vi "N6700_PowerSupplyGUI.vi"(11 "error in (no error)":errorcluster) -> (4 "PsGuiRef":refnum<vi>, 15 "error out":errorcluster {"code" format="%.0x"})   [LabVIEW 2018]
panel:
  out "String":string caption="Timeout"
  in  "Tab Control":enum32{"Page 1", "Page 2"}(tab)
  in  "VISA session":refnum<visa-resource-name>="TCPIP0::169.254.70.130::inst0::INSTR"
  in  "Current Lim":sgl[](array[numeric])
  in  "Voltage Set":sgl[](array[numeric])
  in  "stop":bool=TRUE
  in  "STATE":bool[](array[boolean])=[FALSE, FALSE, FALSE, FALSE]
  out "Volts":dbl[](array[numeric])=[-1.0, -1.0, -1.0, -1.0]
  in  "Measure":bool
  out "Amps":dbl[](array[numeric])=[-1.0, -1.0, -1.0, -1.0]
  in  "RESET_PS":bool=TRUE
  in  "Output Couple Channels(t)":bool=TRUE
  in  "poll rate(ms)":u32=1000
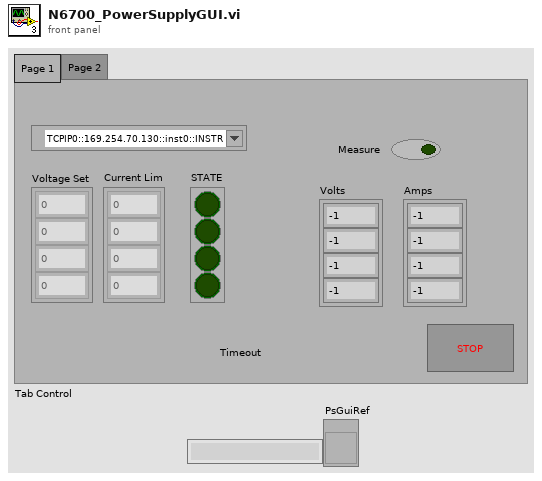
[diagram p1: front panel]
types:
  T1 = enum32{"Invalid", "Standard", "Closed", "Hidden", "Minimized", "Maximized"}
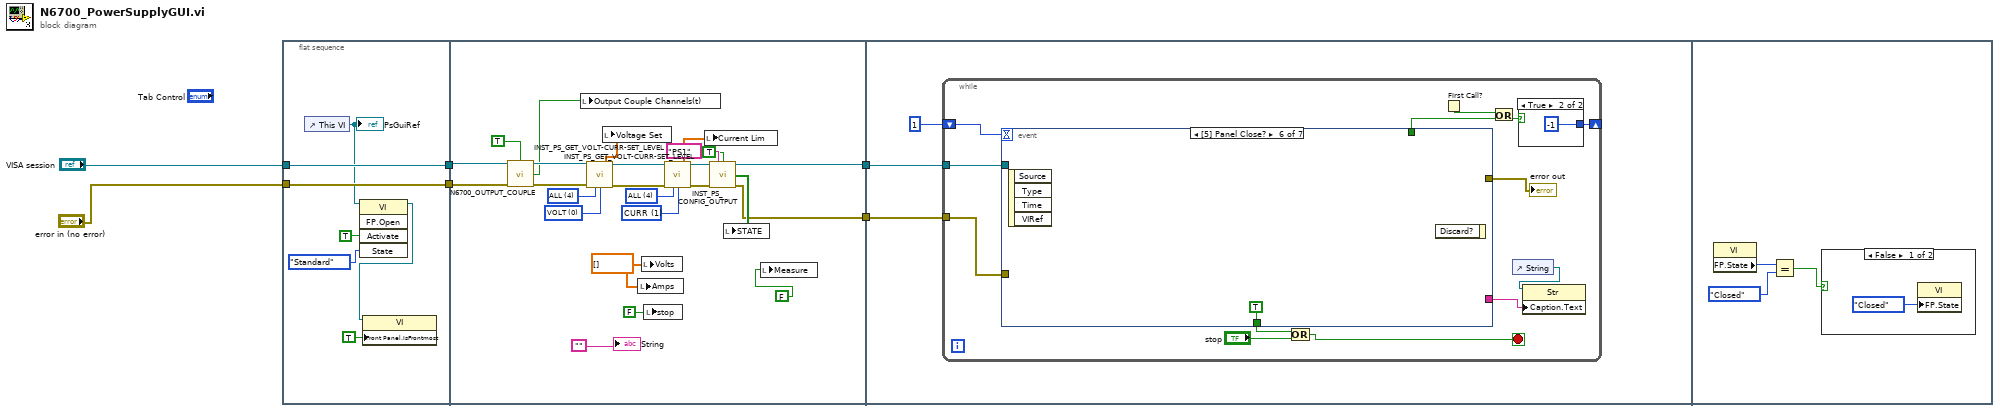
[diagram p0: block diagram]
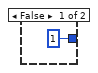
[diagram p2: hidden frame]
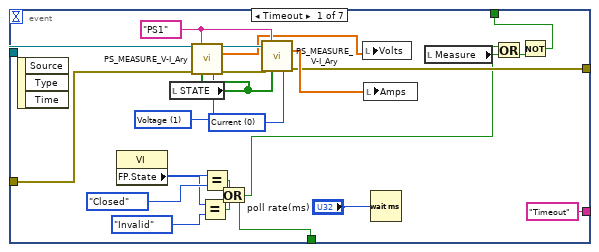
[diagram p3: hidden frame]
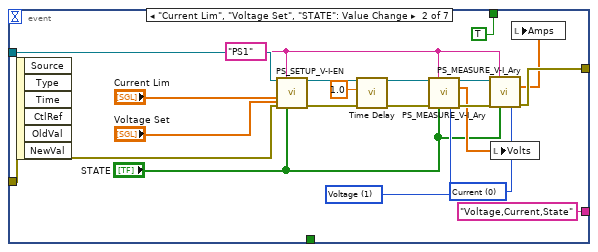
[diagram p4: hidden frame]
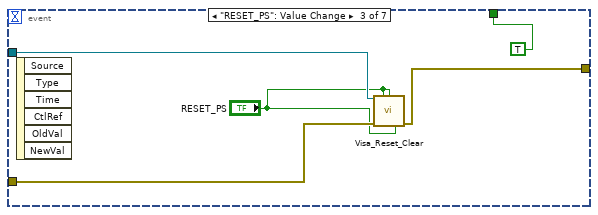
[diagram p5: hidden frame]
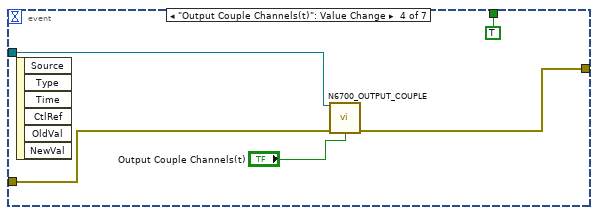
[diagram p6: hidden frame]
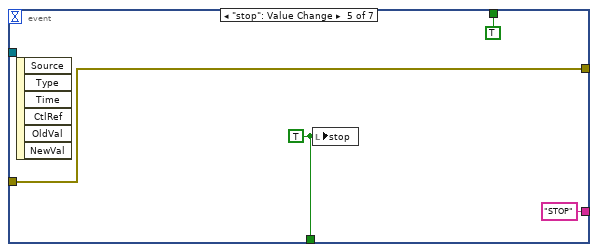
[diagram p7: hidden frame]
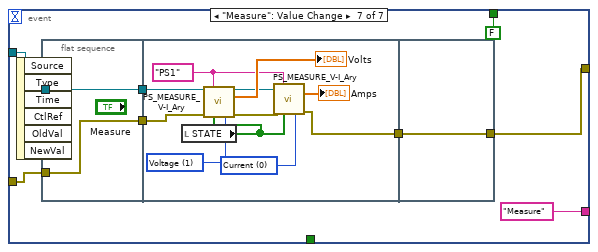
[diagram p8: hidden frame]
diagram:
  n1 = flat-sequence {
    tunnel: "error in (no error)" -> [w12]
    tunnel: "VISA session" -> [w13]
    tunnel: [w13] -> w2
    tunnel: [w12] -> w1
    tunnel: [w24] -> w5
    tunnel: [w21] -> w3
    tunnel: w2 -> [w20]
    tunnel: w1 -> [w19]
    tunnel: w5 -> [w41]
    tunnel: w3 -> [w39]
    frame #0 {
      n2 = control-ref of="This VI"() -> (w11:refnum<vi>)
      "PsGuiRef" <- w11
      n3 = invoke class="VI" method="FP.Open"(reference=w11, "Activate"=TRUE ("Activate?"), "State"=T1."Standard") -> (reference out=w8:refnum<vi>)  [unwired: 2 in, 4 out]
      n4 = property class="VI"(reference=w8, "Front Panel.IsFrontmost"=TRUE ("Front Panel Window:Is Frontmost")) -> ()  [unwired: 1 in, 2 out]
    }
    frame #1 {
      w31 = 0 items=["VOLT", "CURR"] ("V/I")
      w29 = 1 items=["VOLT", "CURR"] ("V/I")
      w30 = 4 items=["1", "2", "3", "4", "ALL"] ("line index")
      w32 = 4 items=["1", "2", "3", "4", "ALL"] ("line index")
      w37 = dbl[] [] ("Volts")
      n5 = call "N6700_OUTPUT_COUPLE.vi"("VISA session"=w20, "RO(T)"=TRUE, "error in (no error)"=w19) -> ("dup VISA session"=w18:refnum<visa-resource-name>, "read_out_coup_on(t)"=w16:bool, "error out"=w17:errorcluster)  [unwired: 10 in]
      n6 = local write "Output Couple Channels(t)"(w16) -> ()
      n7 = call "INST_PS_GET_VOLT-CURR-SET_LEVEL.vi"("VISA session"=w18, "error in (no error)"=w17, "line index"=w32, "V/I"=w31) -> ("Voltage (0.0)"=w33:dbl[], "dup VISA session"=w36:refnum<visa-resource-name>, "error out"=w35:errorcluster)  [unwired: 9 in]
      n8 = local write "Voltage Set"(w33) -> ()
      n9 = local write "Amps"(w37) -> ()
      n10 = local write "Volts"(w37) -> ()
      n11 = local write "stop"(FALSE ("stop")) -> ()
      n12 = call "INST_PS_GET_VOLT-CURR-SET_LEVEL.vi"("VISA session"=w36, "error in (no error)"=w35, "line index"=w30, "V/I"=w29) -> ("Voltage (0.0)"=w34:dbl[], "dup VISA session"=w28:refnum<visa-resource-name>, "error out"=w27:errorcluster)  [unwired: 9 in]
      n13 = local write "Current Lim"(w34) -> ()
      n14 = call "INST_PS_CONFIG_OUTPUT.vi"("VISA session"=w28, "SEL_PS"="PS1", "RO(T)"=TRUE, "error in (no error)"=w27) -> ("dup VISA session"=w24:refnum<visa-resource-name>, "read_out_stat_on(t)"=w23:bool[], "error out"=w21:errorcluster)  [unwired: 9 in]
      n15 = local write "STATE"(w23) -> ()
      n16 = local write "Measure"(FALSE ("Measure")) -> ()
      "String" <- ""
    }
    frame #2 {
      n17 = while {
        tunnel: w41 -> [w54]
        shift-right: [w51] -> _
        shift-left: 1 -> [w53]
        tunnel: w39 -> [w46]
        stop <- w50 stop-if-true
        n18 = event shown="[5] Panel Close?" {
          selector: _ -> [_ _ _ _ _ _ _]
          dyn-events: _ -> [_ _ _ _ _ _ _]
          timeout: w53 -> [_ _ _ _ _ _ _]
          tunnel: w54 -> [w72 w95 w102 w107 _ _ w120]
          tunnel: [w57 _ _ _ w111 TRUE ("stop") _] -> w49
          tunnel: ["Timeout" "Voltage,Current,State" _ _ "STOP" _ "Measure"] -> w47
          tunnel: w46 -> [w68 w93 w101 w105 w109 _ w117]
          tunnel: [w67 w91 w99 w104 w109 _ w115] -> w45
          tunnel: [w64 TRUE TRUE TRUE TRUE _ FALSE] -> w42
          event Timeout {
            w74 = 0 items=["Current", "Voltage"] ("Measurement Type (1: Voltage)")
            w73 = 1 items=["Current", "Voltage"] ("Measurement Type (1: Voltage)")
            w75 = "PS1" ("SEL_PS")
            n19 = event-data() -> ()  [unwired: 1 in, 3 out]
            n20 = property class="VI"() -> ("FP.State"=w60:T1)  [unwired: 2 in, 2 out]
            n21 = local read "STATE"() -> (w76:bool[])
            n22 = call "PS_MEASURE_V-I_Ary.vi"("VISA resource name"=w72, "SEL_PS"=w75, "error in (no error)"=w68, "Array 2"=w76, "Measurement Type (1: Voltage)"=w73) -> ("VISA resource name out"=w78:refnum<visa-resource-name>, "Array"=w71:dbl[], "error out"=w77:errorcluster)  [unwired: 8 in]
            n23 = Equal?(x=w60, y=T1."Invalid" ("Front Panel Window:State")) -> (x = y?=w59:bool)
            n24 = Equal?(x=w60, y=T1."Closed" ("Front Panel Window:State")) -> (x = y?=w62:bool)
            n25 = Or(x=w62, y=w59) -> (x .or. y?=w57:bool)
            n26 = call "PS_MEASURE_V-I_Ary.vi"("VISA resource name"=w78, "SEL_PS"=w75, "error in (no error)"=w77, "Array 2"=w76, "Measurement Type (1: Voltage)"=w74) -> ("Array"=w70:dbl[], "error out"=w67:errorcluster)  [unwired: 8 in, 1 out]
            n27 = local write "Volts"(w71) -> ()
            n28 = local write "Amps"(w70) -> ()
            n29 = Wait (ms)(milliseconds to wait="poll rate(ms)") -> ()  [unwired: 1 out]
            n30 = local read "Measure"() -> (w65:bool)
            n31 = Or(x=w57, y=w65) -> (x .or. y?=w58:bool)
            n32 = Not(x=w58) -> (.not. x?=w64:bool)
          }
          event "Current Lim", "Voltage Set", "STATE": Value Change {
            w85 = 0 items=["Current", "Voltage"] ("Measurement Type (1: Voltage)")
            w86 = 1 items=["Current", "Voltage"] ("Measurement Type (1: Voltage)")
            w88 = "PS1" ("SEL_PS")
            n33 = event-data() -> ()  [unwired: 1 in, 6 out]
            n34 = call "PS_SETUP_V-I-EN.vi"("VISA resource name"=w95, "SEL_PS"=w88, "error in (no error)"=w93, "Use Channel"="STATE", "Current Lim"="Current Lim", "Voltage Set"="Voltage Set") -> ("VISA resource name out"=w90:refnum<visa-resource-name>, "error out"=w81:errorcluster)  [unwired: 8 in]
            n35 = call "Time Delay"("error in (no error)"=w81, "Delay Time (s)"=1.0) -> ("error out"=w82:errorcluster)  [unwired: 9 in]
            n36 = call "PS_MEASURE_V-I_Ary.vi"("VISA resource name"=w90, "SEL_PS"=w88, "error in (no error)"=w82, "Array 2"="STATE", "Measurement Type (1: Voltage)"=w86) -> ("VISA resource name out"=w89:refnum<visa-resource-name>, "Array"=w87:dbl[], "error out"=w92:errorcluster)  [unwired: 8 in]
            n37 = call "PS_MEASURE_V-I_Ary.vi"("VISA resource name"=w89, "SEL_PS"=w88, "error in (no error)"=w92, "Array 2"="STATE", "Measurement Type (1: Voltage)"=w85) -> ("Array"=w84:dbl[], "error out"=w91:errorcluster)  [unwired: 8 in, 1 out]
            n38 = local write "Volts"(w87) -> ()
            n39 = local write "Amps"(w84) -> ()
          }
          event "RESET_PS": Value Change {
            n40 = event-data() -> ()  [unwired: 1 in, 6 out]
            n41 = call "Visa_Reset_Clear.vi"("VISA resource name"=w102, "Send *CLS"="RESET_PS", "Restore Defaults"="RESET_PS", "error in (no error)"=w101, "Send *RST"="RESET_PS") -> ("error out"=w99:errorcluster)  [unwired: 9 in, 1 out]
          }
          event "Output Couple Channels(t)": Value Change {
            n42 = event-data() -> ()  [unwired: 1 in, 6 out]
            n43 = call "N6700_OUTPUT_COUPLE.vi"("VISA session"=w107, "error in (no error)"=w105, "Enable Couple (t)"="Output Couple Channels(t)") -> ("error out"=w104:errorcluster)  [unwired: 10 in, 2 out]
          }
          event "stop": Value Change {
            w111 = TRUE ("stop")
            n44 = event-data() -> ()  [unwired: 1 in, 6 out]
            n45 = local write "stop"(w111) -> ()
          }
          event Panel Close? {
            n46 = event-data() -> ()  [unwired: 1 in, 4 out]
            n47 = event-data() -> ()  [unwired: 2 in, 1 out]
          }
          event "Measure": Value Change {
            n48 = event-data() -> ()  [unwired: 1 in, 6 out]
            n49 = flat-sequence {
              tunnel: w120 -> [w122]
              tunnel: [w122] -> w119
              tunnel: w117 -> [w121]
              tunnel: [w121] -> w116
              tunnel: w119 -> [w132]
              tunnel: w116 -> [w124]
              tunnel: [w123] -> w114
              tunnel: [w134] -> w115
              tunnel: w114 -> [w134]
              frame #0 {
              }
              frame #1 {
                w126 = 0 items=["Current", "Voltage"] ("Measurement Type (1: Voltage)")
                w127 = 1 items=["Current", "Voltage"] ("Measurement Type (1: Voltage)")
                w128 = "PS1" ("SEL_PS")
                n50 = local read "STATE"() -> (w125:bool[])
                n51 = call "PS_MEASURE_V-I_Ary.vi"("VISA resource name"=w132, "SEL_PS"=w128, "error in (no error)"=w124, "Array 2"=w125, "Measurement Type (1: Voltage)"=w127) -> ("VISA resource name out"=w131:refnum<visa-resource-name>, "Array"=→"Volts":dbl[], "error out"=w130:errorcluster)  [unwired: 8 in]
                n52 = call "PS_MEASURE_V-I_Ary.vi"("VISA resource name"=w131, "SEL_PS"=w128, "error in (no error)"=w130, "Array 2"=w125, "Measurement Type (1: Voltage)"=w126) -> ("Array"=→"Amps":dbl[], "error out"=w123:errorcluster)  [unwired: 8 in, 1 out]
              }
              frame #2 {
              }
            }
          }
        }
        "error out" <- w45
        n53 = Or(x=w49, y="stop") -> (x .or. y?=w50:bool)
        n54 = First Call?() -> (First Call?: T/F=w44:bool)
        n55 = Or(x=w44, y=w42) -> (x .or. y?=w43:bool)
        n56 = control-ref of="String"() -> (w48:refnum<vi>)
        n57 = case shown="True" w43 {
          tunnel: [1 -1] -> w51
          frame False {
          }
          frame True {
          }
        }
        n58 = property class="Str"(reference=w48, "Caption.Text"=w47) -> ()  [unwired: 1 in, 2 out]
      }
    }
    frame #3 {
      n59 = property class="VI"() -> ("FP.State"=w136:T1)  [unwired: 2 in, 2 out]
      n60 = Equal?(x=w136, y=T1."Closed" ("Front Panel Window:State")) -> (x = y?=w135:bool)
      n61 = case shown="False" w135 {
        frame False {
          n62 = property class="VI"("FP.State"=T1."Closed" ("Front Panel Window:State")) -> ()  [unwired: 2 in, 2 out]
        }
        frame True {
        }
      }
    }
  }
